vi "Read Channels.vi"(8 "error in (no error)":errorcluster, 11 "Digitizer Instrument in":refnum<class "ACIR Instrument.lvclass">) -> (0 "error out":errorcluster, 2 "Channels":T1[](array[typedef]), 3 "Digitizer Instrument out":refnum<class "ACIR Instrument.lvclass">)   [LabVIEW 2025]
uses:
  ACIR Instrument.lvclass
  Digitizer Dataset.ctl
  ACIR Instrument.lvclass/ACIR Instrument.ctl
  C:/Users/Public/Documents/Sandia National Labs/TSS Plugin/Abstract PlugIn.lvlibp/Plugin/Abstract/Abstract Instrument/Abstract Instrument.lvclass
  C:/Users/Public/Documents/Sandia National Labs/TSS Plugin/CEF.lvlibp/serializable node/CEF_serializable node.lvclass
  C:/Users/Public/Documents/Sandia National Labs/TSS Plugin/CEF.lvlibp/Node/CEF_Node.lvclass
  C:/Working copy/tss/Plugin/Engines/ACIR/ACIR Instrument/ACIR Instrument.lvclass
  C:/Users/Public/Documents/Sandia National Labs/TSS Plugin/Interface.lvlibp/Analog Input/AI.lvclass
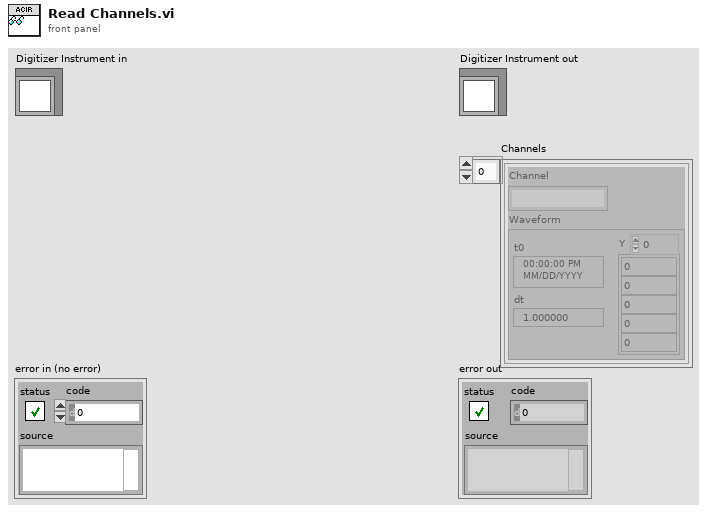
[diagram p1: front panel]
types:
  T1 = typedef "Digitizer Dataset.ctl" = cluster{"Channel":string, "Waveform":waveform(dbl)}
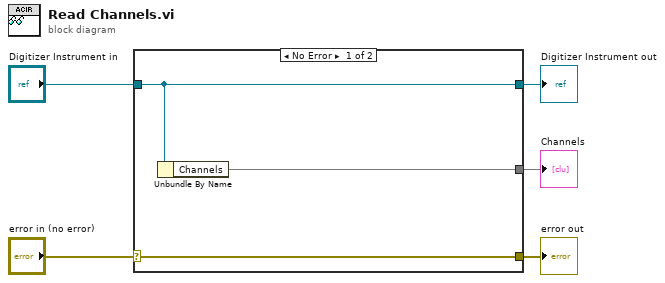
[diagram p0: block diagram]
diagram:
  n1 = case shown="No Error" "error in (no error)" {
    selector: "error in (no error)" -> [w8 w9]
    tunnel: [w8 w9] -> w4
    tunnel: [w7 w10] -> w2
    tunnel: "Digitizer Instrument in" -> [w7 w10]
    tunnel: [w6 _] -> w1
    frame No Error {
      n2 = Unbundle By Name(w7) -> ("Channels"=w6)
    }
    frame Error {
    }
  }
  "error out" <- w4
  "Digitizer Instrument out" <- w2
  "Channels" <- w1
